vi "pp3_log_toString_trial.vi"(8 "input cluster":T1={"Trial Type Number"=1, "Trial Type"=enum."GO", "Trial Weight"=100, "Shock (mA)"=0.3, "Duration (ms)"=250.0, "Sound Type"=enum."04 FM Sweep", "Stim P1"=2000.0, "Stim P2"=4000.0, "Stim P3"=0.0, "Stim P4"=0.0, "DAQ Amplitude (V)"=1.0} {"DAQ Amplitude (V)" min=0.0 max=5.0 format="%_4g"; "Shock (mA)" min=-1.0 max=5.0; "Trial Weight" step=1; "Duration (ms)" min=0.0 max=1.0; "Trial Type Number" min=1 max=256 step=1}, 9 "Run loop diff":i32, 10 "Cum (ms)":i32, 11 "Curr tr":i32) -> (0 "TRIALMEMO String":string, 3 "spreadsheet string":string)   [LabVIEW 2013]
uses:
  pp3_CTL_Trial.ctl
  pp3_CTL_TrialType.ctl
  labolabo2/waveforms/WFTypes.ctl
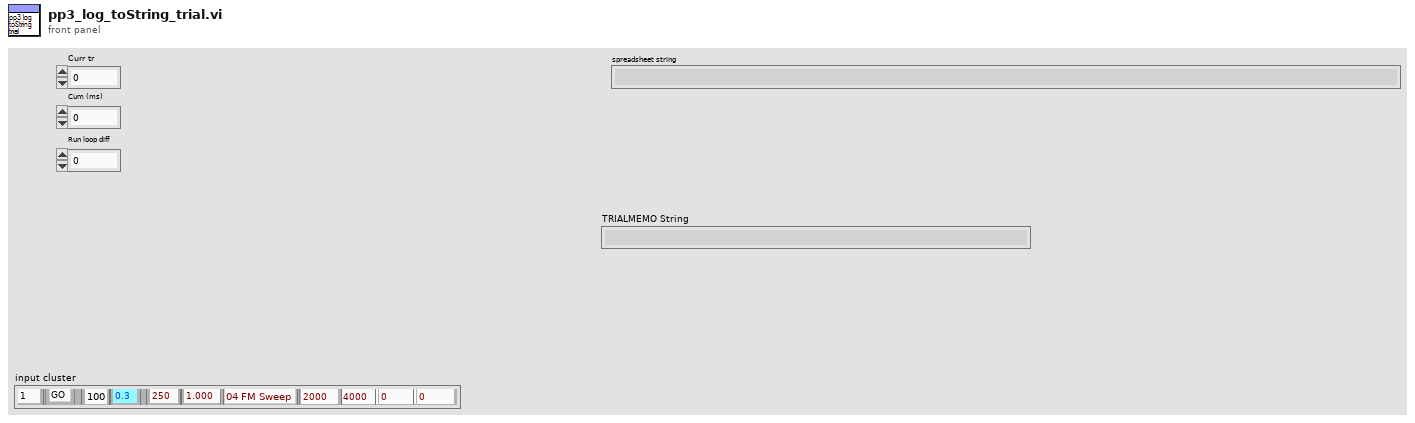
[diagram p1: front panel]
types:
  T1 = typedef "pp3_CTL_Trial.ctl" = cluster{"Trial Type Number":i16, "Trial Type":T2, "Trial Weight":u32, "Shock (mA)":dbl, "Duration (ms)":dbl, "Sound Type":T3, "Stim P1":dbl, "Stim P2":dbl, "Stim P3":dbl, "Stim P4":dbl, "DAQ Amplitude (V)":dbl}
  T2 = typedef "pp3_CTL_TrialType.ctl" = enum16{"OFF", "GO", "NOGO", "TEST"}
  T3 = typedef "WFTypes.ctl" = enum16{"00 NULL", "01 DC", "02 Noise", "03 Pure Tone", "04 FM Sweep"}
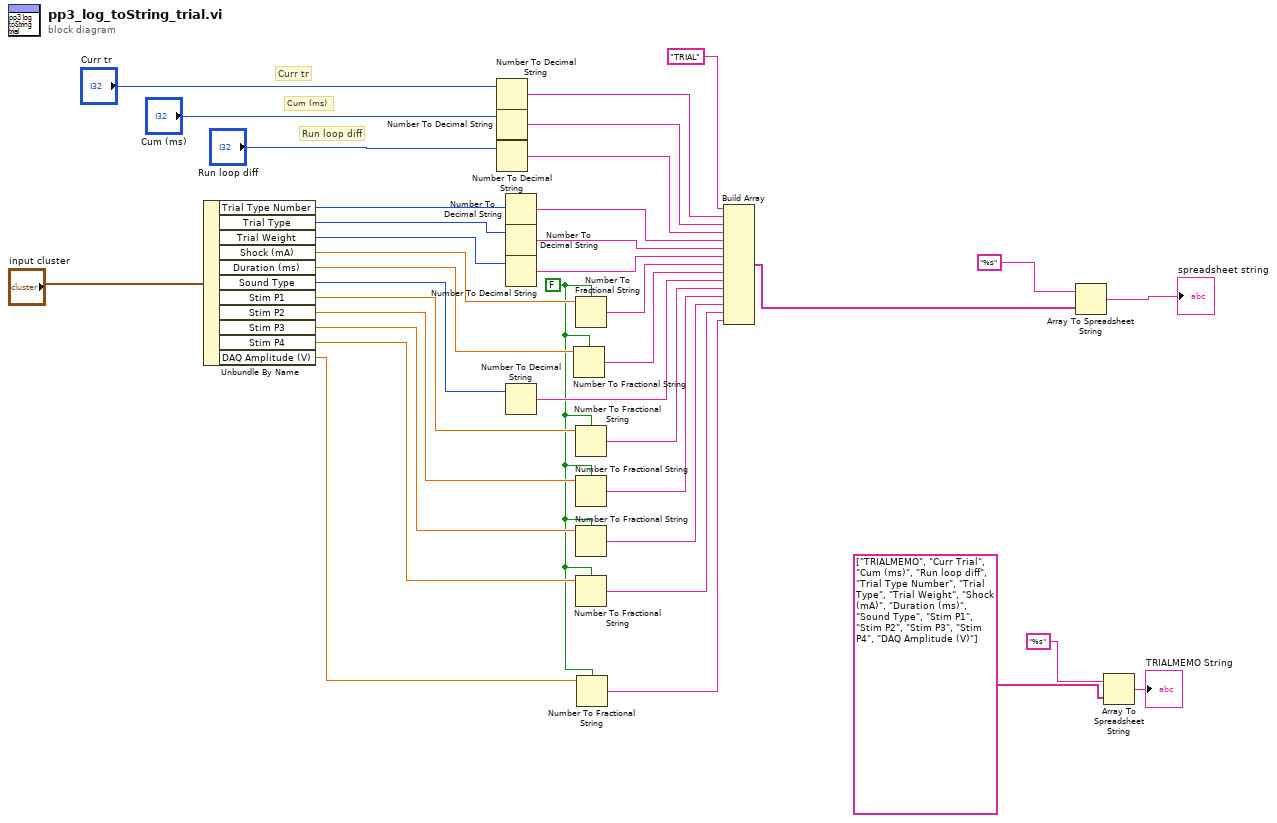
[diagram p0: block diagram]
diagram:
  w7 = FALSE
  # "Run loop diff"
  # "Cum (ms)"
  # "Curr tr"
  n1 = Unbundle By Name("input cluster") -> ("Trial Type Number"=w32:i16, "Trial Type"=w31:T2, "Trial Weight"=w30:u32, "Shock (mA)"=w21:dbl, "Duration (ms)"=w20:dbl, "Sound Type"=w29:T3, "Stim P1"=w19:dbl, "Stim P2"=w18:dbl, "Stim P3"=w17:dbl, "Stim P4"=w16:dbl, "DAQ Amplitude (V)"=w6:dbl)
  n2 = Number To Decimal String(number="Curr tr") -> (decimal integer string=w10:string)  [unwired: 1 in]
  n3 = Number To Decimal String(number="Cum (ms)") -> (decimal integer string=w9:string)  [unwired: 1 in]
  n4 = Number To Decimal String(number="Run loop diff") -> (decimal integer string=w8:string)  [unwired: 1 in]
  n5 = Number To Decimal String(number=w32) -> (decimal integer string=w33:string)  [unwired: 1 in]
  n6 = Number To Decimal String(number=w31) -> (decimal integer string=w37:string)  [unwired: 1 in]
  n7 = Number To Decimal String(number=w30) -> (decimal integer string=w36:string)  [unwired: 1 in]
  n8 = Number To Decimal String(number=w29) -> (decimal integer string=w26:string)  [unwired: 1 in]
  n9 = Number To Fractional String(use system decimal point (T)=w7, number=w20) -> (F-format string=w27:string)  [unwired: 2 in]
  n10 = Number To Fractional String(use system decimal point (T)=w7, number=w21) -> (F-format string=w28:string)  [unwired: 2 in]
  n11 = Number To Fractional String(use system decimal point (T)=w7, number=w19) -> (F-format string=w25:string)  [unwired: 2 in]
  n12 = Number To Fractional String(use system decimal point (T)=w7, number=w18) -> (F-format string=w24:string)  [unwired: 2 in]
  n13 = Number To Fractional String(use system decimal point (T)=w7, number=w17) -> (F-format string=w23:string)  [unwired: 2 in]
  n14 = Number To Fractional String(use system decimal point (T)=w7, number=w16) -> (F-format string=w22:string)  [unwired: 2 in]
  n15 = Number To Fractional String(use system decimal point (T)=w7, number=w6) -> (F-format string=w5:string)  [unwired: 2 in]
  n16 = Build Array("TRIAL" ("element"), w10, w9, w8, w33, w37, w36, w28, w27, w26, w25, w24, w23, w22, w5) -> (w34:string[])
  n17 = Array To Spreadsheet String(array=w34, 3:"%s" ("format string")) -> (spreadsheet string=→"spreadsheet string":string)  [unwired: 1 in]
  n18 = Array To Spreadsheet String(array=string[] ["TRIALMEMO", "Curr Trial", "Cum (ms)", "Run loop diff", "Trial Type Number", "Trial Type", "Trial Weight", "Shock (mA)", "Duration (ms)", "Sound Type", "Stim P1", "Stim P2", "Stim P3", "Stim P4", "DAQ Amplitude (V)"], 3:"%s" ("format string")) -> (spreadsheet string=→"TRIALMEMO String":string)  [unwired: 1 in]
